vi "test Scalar I8.vi"(8 "error in (no error)":errorcluster, 11 "TestCase in":refnum<class "Mem Buff Read Write.lvclass">) -> (0 "error out":errorcluster, 3 "TestCase out":refnum<class "Mem Buff Read Write.lvclass">)   [LabVIEW 2017, in "Mem Buff Read Write.lvclass"]
uses:
  Mem Buff Read Write.lvclass
  Data Sharing Framework Core/Engine/Classes/Buffer/Write 0D I8.vi
  Data Sharing Framework Core/Engine/Classes/Buffer/Read 0D I8.vi
  <vilib>/addons/_JKI Toolkits/VI Tester/TestCase.llb/TestCase.lvclass
  Data Sharing Framework Core/Engine/Classes/Buffer/Buffer.lvclass
  C:/Program Files (x86)/National Instruments/LabVIEW 2017/vi.lib/addons/_JKI Toolkits/VI Tester/TestCase.llb/TestCase.lvclass
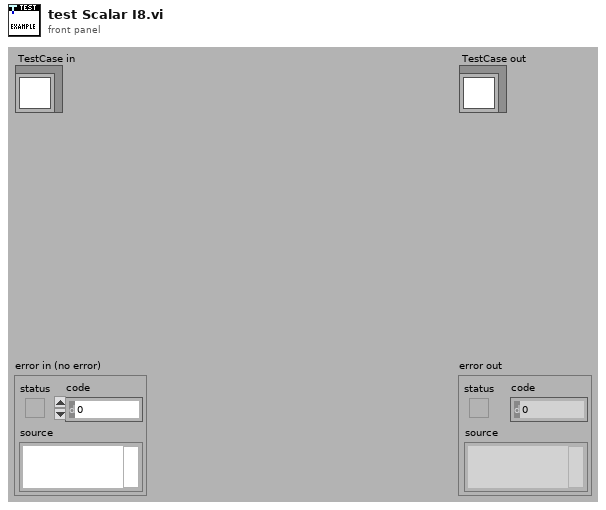
[diagram p1: front panel]
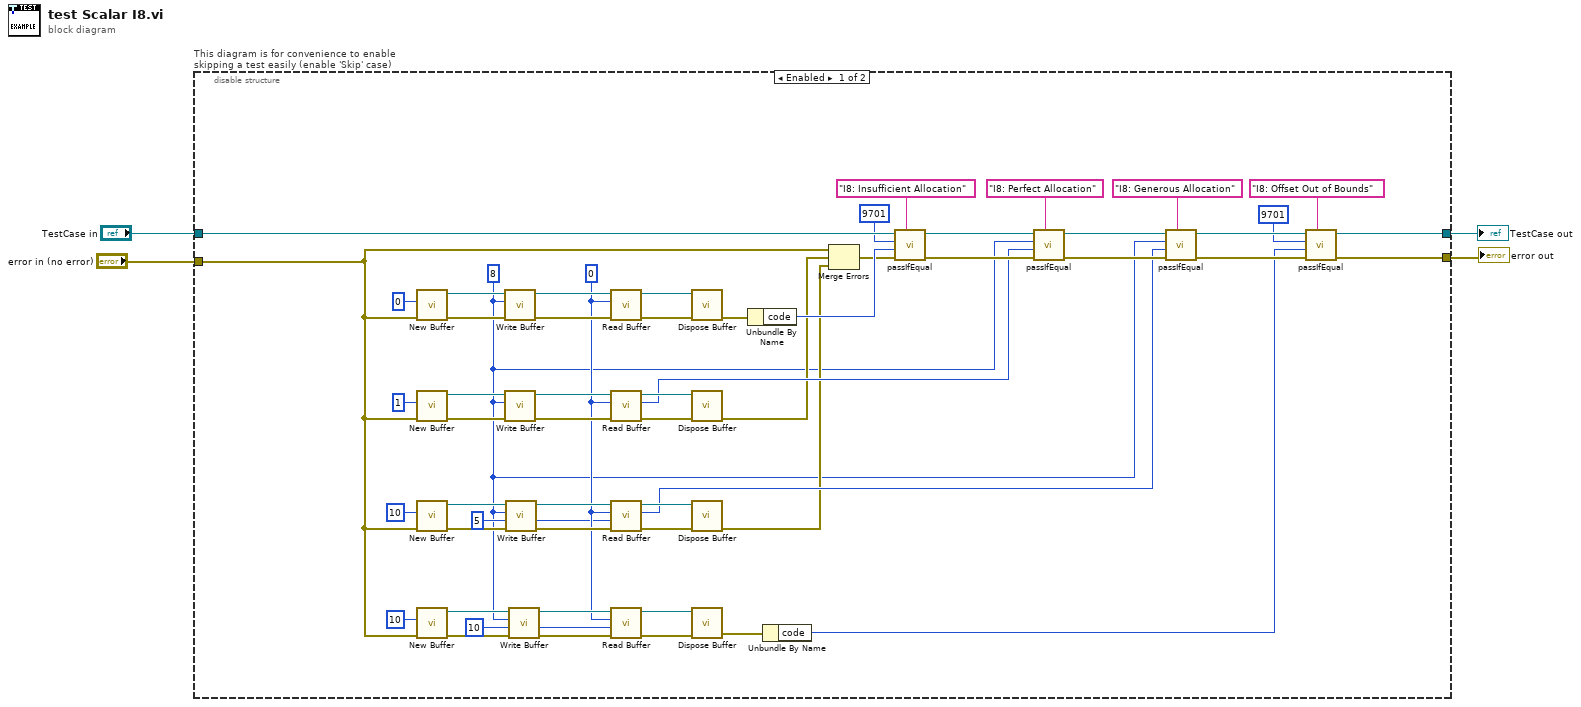
[diagram p0: block diagram]
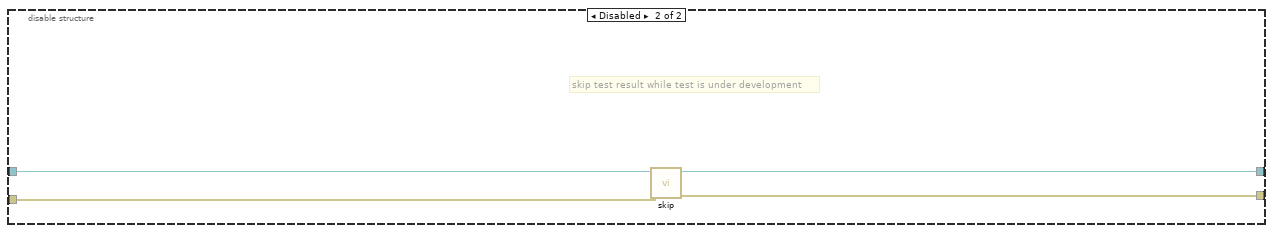
[diagram p2: hidden frame]
diagram:
  n1 = disable-structure "This diagram is for convenience to enable skipping a test easily (enable 'Skip' case)" shown="Enabled" {
    disable-tunnel: "TestCase in" -> [w63 w67]
    disable-tunnel: [w20 w65] -> w1
    disable-tunnel: [w21 w66] -> w3
    disable-tunnel: "error in (no error)" -> [w12 w64]
    frame Enabled {
      w34 = i8 0 ("value in")
      w5 = i8 8 ("value in")
      n2 = call "New Buffer.vi"("error in (no error)"=w12, "size"=u64 0) -> ("error out"=w60:errorcluster, "Buffer out"=w61:refnum<class "Buffer.lvclass">)  [unwired: 8 in]
      n3 = call "New Buffer.vi"("error in (no error)"=w12, "size"=u64 1) -> ("error out"=w51:errorcluster, "Buffer out"=w50:refnum<class "Buffer.lvclass">)  [unwired: 8 in]
      n4 = call "New Buffer.vi"("error in (no error)"=w12, "size"=u64 10) -> ("error out"=w46:errorcluster, "Buffer out"=w47:refnum<class "Buffer.lvclass">)  [unwired: 8 in]
      n5 = call "New Buffer.vi"("error in (no error)"=w12, "size"=u64 10) -> ("error out"=w37:errorcluster, "Buffer out"=w36:refnum<class "Buffer.lvclass">)  [unwired: 8 in]
      n6 = call-poly "Write Buffer.vi"("error in (no error)"=w60, "value in"=w5, "Buffer in"=w61) -> ("error out"=w59:errorcluster, "Buffer out"=w58:refnum<class "Buffer.lvclass">)  [unwired: 5 in, 2 out]
      n7 = call-poly "Write Buffer.vi"("error in (no error)"=w51, "value in"=w5, "Buffer in"=w50) -> ("error out"=w52:errorcluster, "Buffer out"=w53:refnum<class "Buffer.lvclass">)  [unwired: 5 in, 2 out]
      n8 = call-poly "Write Buffer.vi"("error in (no error)"=w46, "offset (0)"=u64 5, "value in"=w5, "Buffer in"=w47) -> ("error out"=w45:errorcluster, "offset out"=w32:u64, "Buffer out"=w44:refnum<class "Buffer.lvclass">)  [unwired: 4 in, 1 out]
      n9 = call-poly "Write Buffer.vi"("error in (no error)"=w37, "offset (0)"=u64 10, "value in"=w5, "Buffer in"=w36) -> ("error out"=w38:errorcluster, "offset out"=w16:u64, "Buffer out"=w39:refnum<class "Buffer.lvclass">)  [unwired: 4 in, 1 out]
      n10 = call-poly "Read Buffer.vi"("error in (no error)"=w59, "value in"=w34, "Buffer in"=w58) -> ("error out"=w57:errorcluster, "Buffer out"=w31:refnum<class "Buffer.lvclass">)  [unwired: 5 in, 2 out]
      n11 = call-poly "Read Buffer.vi"("error in (no error)"=w52, "value in"=w34, "Buffer in"=w53) -> ("error out"=w55:errorcluster, "value out"=w26:i8, "Buffer out"=w54:refnum<class "Buffer.lvclass">)  [unwired: 5 in, 1 out]
      n12 = call-poly "Read Buffer.vi"("error in (no error)"=w45, "offset (0)"=w32, "value in"=w34, "Buffer in"=w44) -> ("error out"=w42:errorcluster, "value out"=w19:i8, "Buffer out"=w43:refnum<class "Buffer.lvclass">)  [unwired: 4 in, 1 out]
      n13 = call-poly "Read Buffer.vi"("error in (no error)"=w38, "offset (0)"=w16, "value in"=w34, "Buffer in"=w39) -> ("error out"=w41:errorcluster, "Buffer out"=w40:refnum<class "Buffer.lvclass">)  [unwired: 4 in, 2 out]
      n14 = call "Dispose Buffer.vi"("error in (no error)"=w57, "Buffer in"=w31) -> ("error out"=w29:errorcluster)  [unwired: 9 in]
      n15 = call "Dispose Buffer.vi"("error in (no error)"=w55, "Buffer in"=w54) -> ("error out"=w11:errorcluster)  [unwired: 9 in]
      n16 = call "Dispose Buffer.vi"("error in (no error)"=w42, "Buffer in"=w43) -> ("error out"=w10:errorcluster)  [unwired: 9 in]
      n17 = call "Dispose Buffer.vi"("error in (no error)"=w41, "Buffer in"=w40) -> ("error out"=w18:errorcluster)  [unwired: 9 in]
      n18 = Unbundle By Name(w29) -> ("code"=w27:i32)
      n19 = Unbundle By Name(w18) -> ("code"=w15:i32)
      n20 = Merge Errors(w12, w11, w10) -> (w13:errorcluster)
      n21 = call-dynamic "passIfEqual.vi"("custom report message (\"\")"="I8: Insufficient Allocation" ("custom report message (\"\")"), "error in (no error)"=w13, "y"=w27, "x"=9701 ("code"), "TestCase in"=w63) -> ("error out"=w30:errorcluster, "TestCase out"=w56:refnum<class "Mem Buff Read Write.lvclass">)  [unwired: 5 in]
      n22 = call-dynamic "passIfEqual.vi"("custom report message (\"\")"="I8: Perfect Allocation" ("custom report message (\"\")"), "error in (no error)"=w30, "y"=w26, "x"=w5, "TestCase in"=w56) -> ("error out"=w23:errorcluster, "TestCase out"=w25:refnum<class "Mem Buff Read Write.lvclass">)  [unwired: 5 in]
      n23 = call-dynamic "passIfEqual.vi"("custom report message (\"\")"="I8: Generous Allocation" ("custom report message (\"\")"), "error in (no error)"=w23, "y"=w19, "x"=w5, "TestCase in"=w25) -> ("error out"=w22:errorcluster, "TestCase out"=w24:refnum<class "Mem Buff Read Write.lvclass">)  [unwired: 5 in]
      n24 = call-dynamic "passIfEqual.vi"("custom report message (\"\")"="I8: Offset Out of Bounds" ("custom report message (\"\")"), "error in (no error)"=w22, "y"=w15, "x"=9701 ("code"), "TestCase in"=w24) -> ("error out"=w21:errorcluster, "TestCase out"=w20:refnum<class "Mem Buff Read Write.lvclass">)  [unwired: 5 in]
    }
    frame Disabled {
      # "skip test result while test is under development"
      n25 = call <vilib>:"skip.vi"("error in (no error)"=w64, "TestCase in"=w67) -> ("error out"=w66:errorcluster, "TestCase out"=w65:refnum<class "Mem Buff Read Write.lvclass">)  [unwired: 8 in]
    }
  }
  "error out" <- w3
  "TestCase out" <- w1
